vi "Write OPC UA Client Refnum.vi"(8 "error in (no error)":errorcluster, 10 "Server Connection Information.Server Endpoint URL":string, 11 "UA Server in":refnum<class "UA Server.lvclass">) -> (0 "error out":errorcluster, 3 "UA Server out":refnum<class "UA Server.lvclass">)   [LabVIEW 2017, in "opcua.lvlib" / "Browser Core.lvlib" / "UA Server.lvclass"]
uses:
  UA Server.lvclass
  UA Server.lvclass/UA Server.ctl
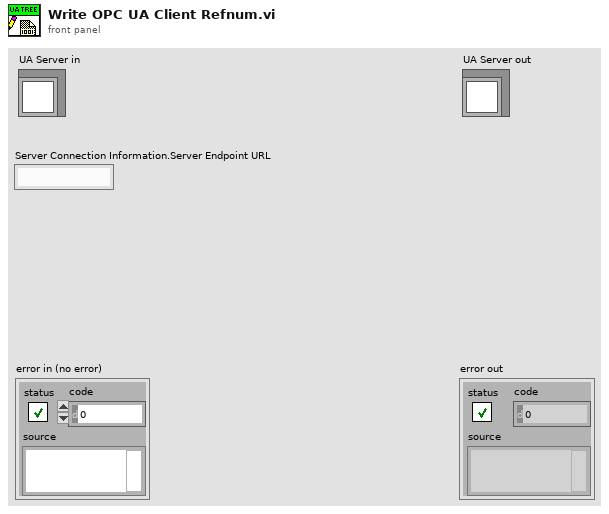
[diagram p1: front panel]
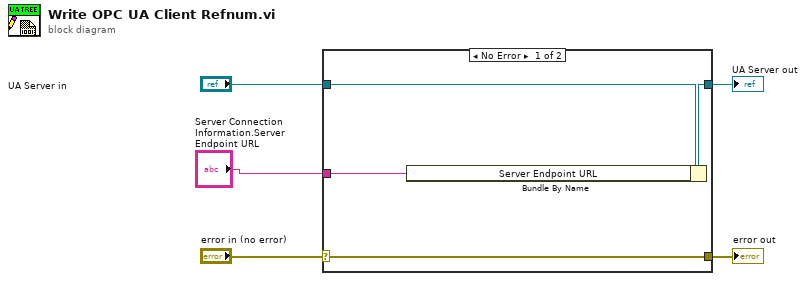
[diagram p0: block diagram]
diagram:
  n1 = case shown="No Error" "error in (no error)" {
    selector: "error in (no error)" -> [w9 w10]
    tunnel: [w9 w10] -> w4
    tunnel: [w7 w11] -> w2
    tunnel: "UA Server in" -> [w8 w11]
    tunnel: "Server Connection Information.Server Endpoint URL" -> [w6 _]
    frame No Error {
      n2 = Bundle By Name(cluster=w8, "Server Endpoint URL"=w6) -> (w7:refnum<class "UA Server.lvclass">)
    }
    frame Error {
    }
  }
  "error out" <- w4
  "UA Server out" <- w2
